vi "Initialise.vi"(8 "error in (no error)":errorcluster, 10 "Message in":refnum<class "InitialiseMessage.lvclass">, 11 "BMC in":refnum<class "BMC.lvclass">) -> (0 "error out":errorcluster, 3 "BMC out":refnum<class "BMC.lvclass">)   [LabVIEW 2012, in "BMC.lvclass"]
doc: "This method is called when an initialise message is received. It mainly initialises the RabbitMQ connectivity. \n\nOverride this method when your component needs special initialisation (e.g. of software or hardware resources). In that case, don't forget to call the parent for proper implementation. If your component owns subcomponents, they count as resources, so you have to initialise them by calling their own initialise functions"
uses:
  BMC.lvclass
  <vilib>/Distrio/Murmex/InitialiseMessage/InitialiseMessage.lvclass
  <vilib>/Distrio/Murmex/Murmex/Murmex.lvclass
  BMC.lvclass/BMC.ctl
panel:
  # "This method is called when the INTIALISE\ntrigger is sent. \n\nOverride this method when your component needs to\nrespond to this trigger. \n\nCall parent for proper implementation"
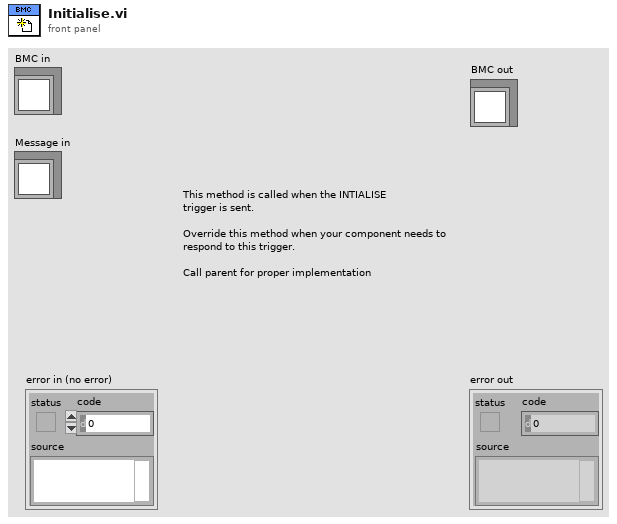
[diagram p1: front panel]
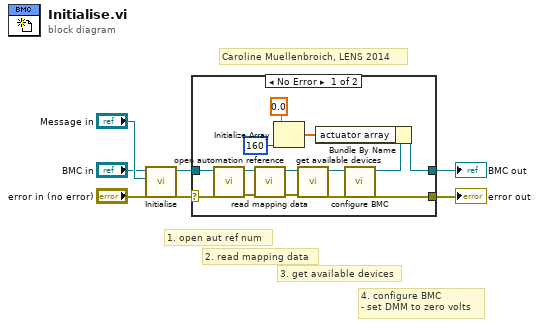
[diagram p0: block diagram]
diagram:
  # "2. read mapping data"
  # "4. configure BMC\n- set DMM to zero volts"
  # "Caroline Muellenbroich, LENS 2014"
  # "3. get available devices"
  # "1. open aut ref num"
  n1 = call-parent "Initialise.vi"("error in (no error)"="error in (no error)", "Message in"="Message in", "Murmex in"="BMC in") -> ("error out"=w4:errorcluster, "Murmex out"=w2:refnum<class "BMC.lvclass">)  [unwired: 7 in]
  n2 = case shown="No Error" w4 {
    selector: w4 -> [w21 w23]
    tunnel: [w18 w23] -> w3
    tunnel: w2 -> [w13 w22]
    tunnel: [w11 w22] -> w1
    frame No Error {
      n3 = call-dynamic "open automation reference.vi"("error in (no error)"=w21, "BMC in"=w13) -> ("error out"=w15:errorcluster, "BMC out"=w17:refnum<class "BMC.lvclass">)  [unwired: 8 in]
      n4 = call-dynamic "read mapping data.vi"("error in (no error)"=w15, "BMC in"=w17) -> ("error out"=w14:errorcluster, "BMC out"=w16:refnum<class "BMC.lvclass">)  [unwired: 8 in]
      n5 = Initialize Array(0.0 ("element"), 160 ("dimension size")) -> (w10:dbl[])
      n6 = call-dynamic "get available devices.vi"("error in (no error)"=w14, "BMC in"=w16) -> ("error out"=w20:errorcluster, "BMC out"=w19:refnum<class "BMC.lvclass">)  [unwired: 8 in]
      n7 = call-dynamic "configure BMC.vi"("error in (no error)"=w20, "BMC in"=w19) -> ("error out"=w18:errorcluster, "BMC out"=w12:refnum<class "BMC.lvclass">)  [unwired: 8 in]
      n8 = Bundle By Name(cluster=w12, "actuator array"=w10) -> (w11:refnum<class "BMC.lvclass">)
    }
    frame Error {
    }
  }
  "error out" <- w3
  "BMC out" <- w1
